vi "Begin.vi"(8 "error in":errorcluster) -> (0 "error out":errorcluster)   [LabVIEW 2015]
doc: "Called before other user functions, this VI is expected to open initial I/O refnums, load in file data, and do all program initialization. Notice that the <B>error out</B> terminal is simply used for data flow. Wiring it to other structures or subVIs ensures that this VI runs first."
uses:
  <vilib>/Rock Robotics/SystemInterfaces/DIO/FPGA_DIOPWMChannel.ctl
  <vilib>/Rock Robotics/WPI/SafetyOutput/WPI_SafetyOutputConfigMenu.ctl
  <vilib>/Rock Robotics/WPI/DriverStation/WPI_DriverStationRobotMode2.ctl
  <vilib>/Rock Robotics/WPI/Joystick/WPI_JoystickDeviceEnum.ctl
  <vilib>/Rock Robotics/SystemInterfaces/DIO/FPGA_DIOChannel.ctl
  <vilib>/Rock Robotics/WPI/Solenoid/WPI_SolenoidChannel.ctl
  <vilib>/Rock Robotics/WPI/RobotDrive/WPI_RobotDriveOpen2MotorWithVictorSP.vi
  Robot Global Data.vi
  <vilib>/Rock Robotics/Network Tables/SD Write String Array.vi
  Globals.vi
  <vilib>/Rock Robotics/WPI/MotorControl/WPI_MotorControlOpen VictorSP.vi
  <vilib>/Rock Robotics/WPI/Solenoid/WPI_SolenoidOpenDouble.vi
  <vilib>/Rock Robotics/WPI/Utilities/WPI_GetSetVariantRefNum.vi
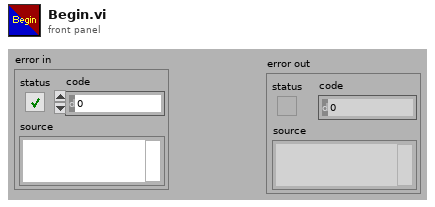
[diagram p1: front panel]
types:
  T1 = typedef "FPGA_DIOPWMChannel.ctl" = enum8{"PWM 0", "PWM 1", "PWM 2", "PWM 3", "PWM 4", "PWM 5", "PWM 6", "PWM 7", "PWM 8", "PWM 9", "PWM MXP 0", "PWM MXP 1", "PWM MXP 2", "PWM MXP 3", "PWM MXP 4", "PWM MXP 5", "PWM MXP 6", "PWM MXP 7", "PWM MXP 8", "PWM MXP 9", "Invalid"}
  T2 = typedef "WPI_SolenoidChannel.ctl" = enum8{"Solenoid 0", "Solenoid 1", "Solenoid 2", "Solenoid 3", "Solenoid 4", "Solenoid 5", "Solenoid 6", "Solenoid 7", "Invalid"}
  T3 = typedef "FPGA_DIOChannel.ctl" = enum8{"DIO 0", "DIO 1", "DIO 2", "DIO 3", "DIO 4", "DIO 5", "DIO 6", "DIO 7", "DIO 8", "DIO 9", "DIO MXP 0", "DIO MXP 1", "DIO MXP 2", "DIO MXP 3", "DIO MXP 4", "DIO MXP 5", "DIO MXP 6", "DIO MXP 7", "DIO MXP 8", "DIO MXP 9", "DIO MXP 10", "DIO MXP 11", "DIO MXP 12", "DIO MXP 13", "DIO MXP 14", "DIO MXP 15", "Invalid"}
  T4 = typedef "WPI_JoystickDeviceEnum.ctl" = enum16{"USB 0", "USB 1", "USB 2", "USB 3", "USB 4", "USB 5"}
  T5 = typedef "WPI_DriverStationRobotMode2.ctl" = enum16{"Autonomous Disabled", "Autonomous Enabled", "Teleop Disabled", "Teleop Enabled", "Disconnected", "Finish", "Test Disabled", "Test Enabled", "Emergency Stopped"}
  T6 = typedef "WPI_SafetyOutputConfigMenu.ctl" = enum16{"Enable", "Disable"}
  T7 = typedef "WPI_JoystickDevRef.ctl" = cluster{"Device":T4}
  T8 = typedef "WPI_RobotDriveDevRef.ctl" = cluster{"DevStatus":errorcluster, "Motors[]":T9[], "Square Inputs":bool, "Max Output":dbl}
  T9 = typedef "WPI_MotorControlDeviceRef.ctl" = cluster{"DeviceStatus":errorcluster, "Type":T10, "PWM":cluster{"PWM Channel":T1, "DeadBand":T11}, "CAN":cluster{"Device Number":u8, "Control Mode":T12, "Semaphore":T13, "Max Vout":dbl, "TalonSRX Control Mode":T14}, "Invert":bool}
  T10 = typedef "WPI_MotorControlType.ctl" = enum16{"PWM", "CAN", "CANTalonSRX"}
  T11 = typedef "WPI_PWMDeadband.ctl" = cluster{"Name":string, "maxPositivePwm":i32, "minPositivePwm":i32, "centerPwm":i32, "maxNegativePwm":i32, "minNegativePwm":i32, "angularRange":u16}
  T12 = typedef "WPI_CANJaguar_ControlMode.ctl" = enum8{"Percent VBus", "Current", "Speed", "Position", "Voltage"}
  T13 = typedef "Semaphore RefNum" = refnum<k1>
  T14 = typedef "WPI_CANTalonSRX_APIControlMode.ctl" = enum8{"Percent VBus", "Speed", "Position", "Slave", "Unchanged / Invalid", "Voltage Compensation", "Current", "Motion Profile"}
  T15 = typedef "WPI_CompressorDevRef.ctl" = cluster{"DevStatus":errorcluster, "Pneumatics Control Module":u8}
  T16 = typedef "WPI_SolenoidDevRef.ctl" = cluster{"DevStatus":errorcluster, "Pneumatics Control Module":u8, "Forward Solenoid Channel":T2, "Reverse Solenoid Channel":T2}
  T17 = typedef "WPI_DigitalInputDevRef.ctl" = cluster{"DevStatus":errorcluster, "DIO Channel":T3}
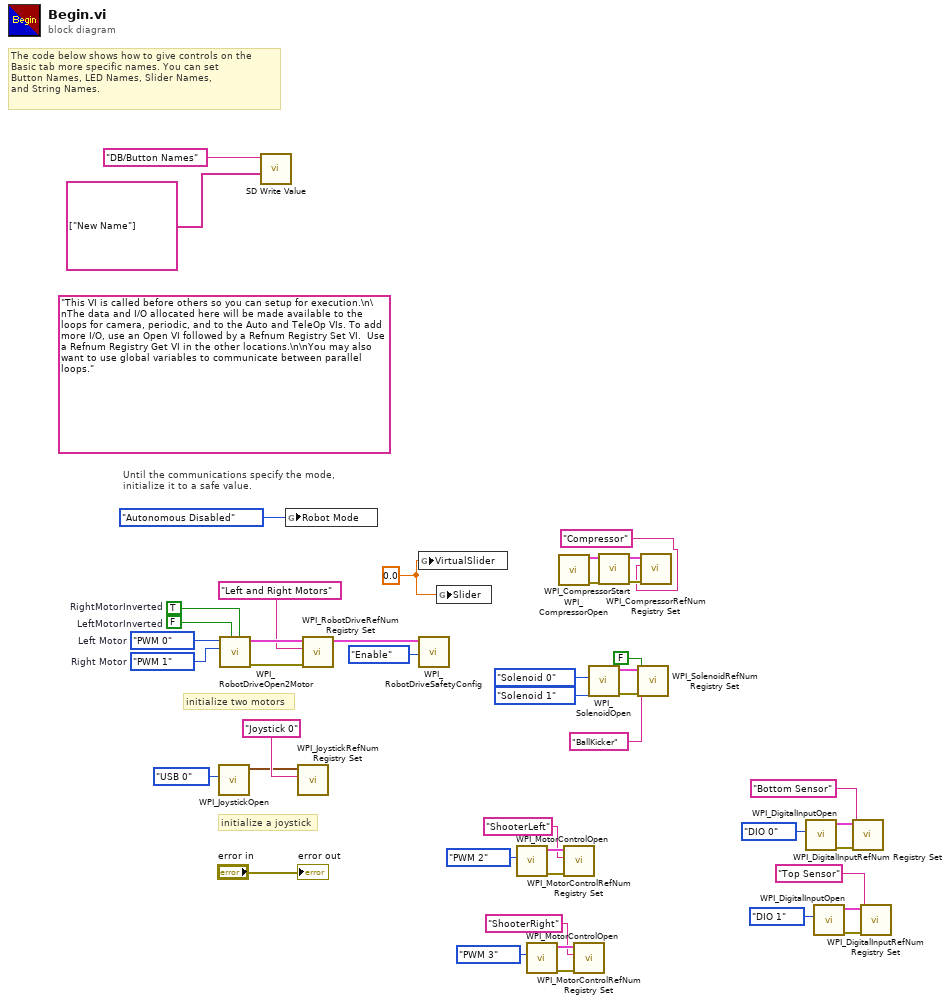
[diagram p0: block diagram]
diagram:
  w30 = 0.0
  (unwired) "This VI is called before others so you can setup for execution.\n\nThe data and I/O allocated here will be made available to the loops for camera, periodic, and to the Auto and TeleOp VIs. To add more I/O, use an Open VI followed by a Refnum Registry Set VI.  Use a Refnum Registry Get VI in the other locations.\n\nYou may also want to use global variables to communicate between parallel loops."
  w39 = FPGA_DIOPWMChannel."PWM 1"  # Right Motor
  w40 = FPGA_DIOPWMChannel."PWM 0"  # Left Motor
  w43 = FALSE  # LeftMotorInverted
  w44 = TRUE  # RightMotorInverted
  # "The code below shows how to give controls on the\nBasic tab more specific names. You can set\nButton Names, LED Names, Slider Names,\nand String Names."
  # "initialize a joystick"
  # "Until the communications specify the mode,\ninitialize it to a safe value."
  # "initialize two motors"
  n1 = call <vilib>:"WPI_JoystickOpen.vi"("JoystickDevice"=WPI_JoystickDeviceEnum."USB 0") -> ("JoystickDevRef"=w35:T7)  [unwired: 10 in]
  n2 = call-poly <vilib>:"WPI_RobotDriveOpen2Motor.vi"("Right Motor Inverted"=w44, "Left Motor Inverted"=w43, "Right Motor"=w39, "Left Motor"=w40) -> ("error out"=w28:errorcluster, "RobotDriveDevRef"=w42:T8)  [unwired: 1 in, 5 out]
  n3 = call-poly <vilib>:"SD Write Value.vi"("String Array"=string[] ["New Name"], "Name"="DB/Button Names") -> ()  [unwired: 8 in, 2 out]
  n4 = global write "Robot Global Data.vi" "Robot Mode"(WPI_DriverStationRobotMode2."Autonomous Disabled" ("Robot Mode")) -> ()
  n5 = call <vilib>:"WPI_JoystickRefNum Registry Set.vi"("refnum name"="Joystick 0", "JoystickDevRef"=w35) -> ()  [unwired: 8 in, 2 out]
  n6 = call <vilib>:"WPI_RobotDriveRefNum Registry Set.vi"("error in (no error)"=w28, "refnum name"="Left and Right Motors", "RobotDriveDevRef"=w42) -> ("RobotDriveDevRef"=w29:T8)  [unwired: 1 in, 7 out]
  n7 = global write "Globals.vi" "VirtualSlider"(w30) -> ()
  n8 = call <vilib>:"WPI_RobotDriveSafetyConfig.vi"("mode"=WPI_SafetyOutputConfigMenu."Enable", "RobotDriveDevRef"=w29) -> ()  [unwired: 8 in, 2 out]
  n9 = global write "Globals.vi" "Slider"(w30) -> ()
  n10 = call-poly <vilib>:"WPI_MotorControlOpen.vi"("PWM Channel"=FPGA_DIOPWMChannel."PWM 2") -> ("error out"=w26:errorcluster, "MotorControlDeviceRef"=w25:T9)  [unwired: 9 in]
  n11 = call-poly <vilib>:"WPI_MotorControlOpen.vi"("PWM Channel"=FPGA_DIOPWMChannel."PWM 3") -> ("error out"=w3:errorcluster, "MotorControlDeviceRef"=w2:T9)  [unwired: 9 in]
  n12 = call <vilib>:"WPI_CompressorOpen.vi"() -> ("CompressorDevRef"=w14:T15, "error out"=w15:errorcluster)  [unwired: 14 in]
  n13 = call <vilib>:"WPI_MotorControlRefNum Registry Set.vi"("error in (no error)"=w26, "refnum name"="ShooterLeft", "MotorControlDevRef"=w25) -> ()  [unwired: 7 in, 2 out]
  n14 = call <vilib>:"WPI_MotorControlRefNum Registry Set.vi"("error in (no error)"=w3, "refnum name"="ShooterRight", "MotorControlDevRef"=w2) -> ()  [unwired: 7 in, 2 out]
  n15 = call-poly <vilib>:"WPI_SolenoidOpen.vi"("Reverse Solenoid Channel"=WPI_SolenoidChannel."Solenoid 1", "Forward Solenoid Channel"=WPI_SolenoidChannel."Solenoid 0") -> ("error out"=w10:errorcluster, "SolenoidDevRef"=w9:T16)  [unwired: 8 in]
  n16 = call <vilib>:"WPI_CompressorStart.vi"("error in (no error)"=w15, "CompressorDevRef"=w14) -> ("error out"=w13:errorcluster, "CompressorDevRef"=w12:T15)  [unwired: 8 in]
  n17 = call <vilib>:"WPI_SolenoidRefNum Registry Set.vi"("error in (no error)"=w10, "Test Mode Only"=FALSE, "refnum name"="BallKicker", "SolenoidDevRef"=w9) -> ()  [unwired: 6 in, 2 out]
  n18 = call <vilib>:"WPI_CompressorRefNum Registry Set.vi"("error in (no error)"=w13, "refnum name"="Compressor", "CompressorDevRef"=w12) -> ()  [unwired: 7 in, 2 out]
  n19 = call <vilib>:"WPI_DigitalInputOpen.vi"("DIO Channel"=FPGA_DIOChannel."DIO 0") -> ("error out"=w22:errorcluster, "DigitalInputDevRef"=w21:T17)  [unwired: 9 in]
  n20 = call <vilib>:"WPI_DigitalInputOpen.vi"("DIO Channel"=FPGA_DIOChannel."DIO 1") -> ("error out"=w18:errorcluster, "DigitalInputDevRef"=w17:T17)  [unwired: 9 in]
  n21 = call <vilib>:"WPI_DigitalInputRefNum Registry Set.vi"("error in (no error)"=w22, "refnum name"="Bottom Sensor", "DigitalInputDevRef"=w21) -> ()  [unwired: 7 in, 2 out]
  n22 = call <vilib>:"WPI_DigitalInputRefNum Registry Set.vi"("error in (no error)"=w18, "refnum name"="Top Sensor", "DigitalInputDevRef"=w17) -> ()  [unwired: 7 in, 2 out]
  "error out" <- "error in"
